vi "RST_XDM3051.vi"(8 "error in":errorcluster, 11 "RS232_Input":refnum<visa-resource-name>) -> (0 "error out":errorcluster, 2 "response":string, 3 "RS232_Output":refnum<visa-resource-name>)   [LabVIEW 2017]
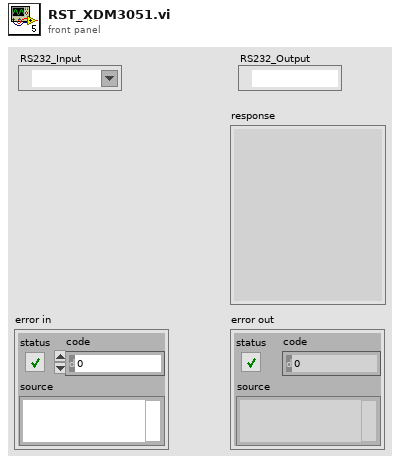
[diagram p1: front panel]
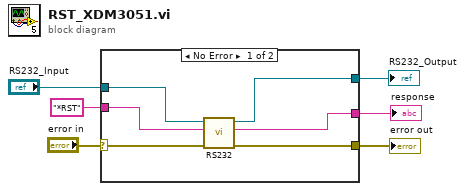
[diagram p0: block diagram]
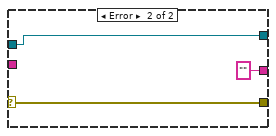
[diagram p2: hidden frame]
diagram:
  n1 = case shown="No Error" "error in" {
    selector: "error in" -> [w12 w15]
    tunnel: [w11 w15] -> w5
    tunnel: "RS232_Input" -> [w10 w14]
    tunnel: "*RST" ("command") -> [w9 _]
    tunnel: [w8 "" ("response")] -> w2
    tunnel: [w7 w14] -> w1
    frame No Error {
      n2 = call "RS232.vi"("error in"=w12, "command"=w9, "RS232_Input"=w10) -> ("error out"=w11:errorcluster, "response"=w8:string, "RS232_Output"=w7:refnum<visa-resource-name>)  [unwired: 6 in]
    }
    frame Error {
    }
  }
  "error out" <- w5
  "RS232_Output" <- w1
  "response" <- w2
